vi "Project Documentation 2012 NIVerified.vi"() -> ()   [LabVIEW 2021]
panel:
  out "Project Descriptions":string[](array[string])
  # "Overview: This example uses recursion to harvest and publish documentation for a LabVIEW project.\nRequirements: LabVIEW 2012 (or compatible)\nInstructions:\n1. Open the project(s) you want to document.\n2. Run this VI .\n3. Observe the  Project Descriptions control, it will document all the open projects, and change the index to see\n documentation of different projects."
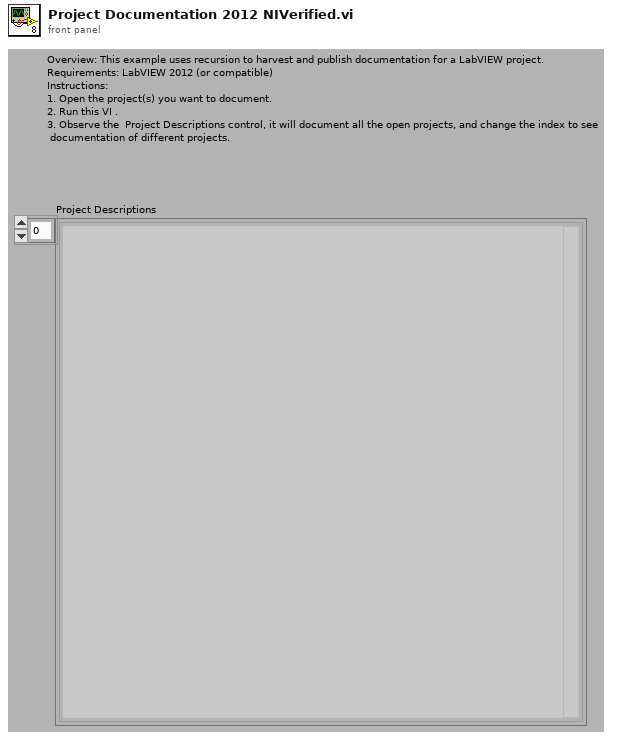
[diagram p1: front panel]
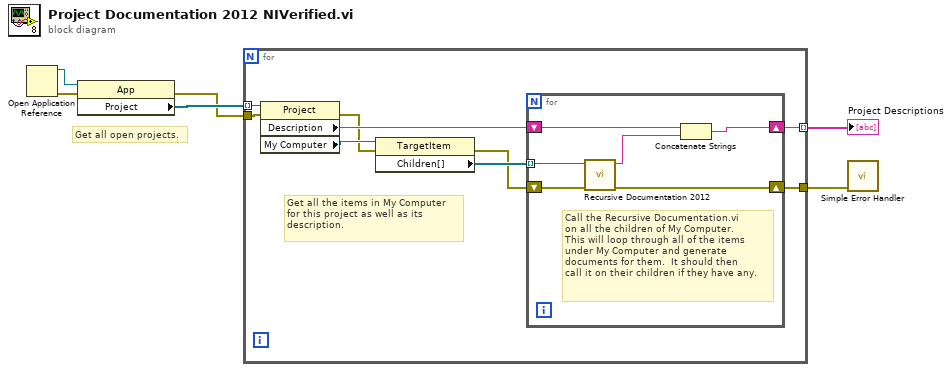
[diagram p0: block diagram]
diagram:
  # "Get all open projects."
  n1 = Open Application Reference() -> (0:w5:errorcluster, 3:w6:refnum<vi>)  [unwired: 4 in]
  n2 = property class="App"(reference=w6, error in=w5) -> (error out=w2:errorcluster, "Project"=w4:refnum<vi>[])  [unwired: 1 out]
  n3 = for {
    tunnel: w4 -> [w11] mode=indexing
    tunnel: [w12] -> w3 mode=indexing
    tunnel: w2 -> [w10]
    tunnel: [w7] -> w1
    # "Get all the items in My Computer\nfor this project as well as its\ndescription."
    n4 = property class="Project"(reference=w11, error in=w10) -> (error out=w9:errorcluster, "Description"=w13:string, "My Computer"=w15:refnum<vi>)  [unwired: 1 out]
    n5 = property class="TargetItem"(reference=w15, error in=w9) -> (error out=w8:errorcluster, "Children[]"=w14:refnum<vi>[])  [unwired: 1 out]
    n6 = for {
      tunnel: w14 -> [w21] mode=indexing
      shift-right: [w18] -> w12
      shift-left: w13 -> [w19]
      shift-right: [w16] -> w7
      shift-left: w8 -> [w20]
      # "Call the Recursive Documentation.vi \non all the children of My Computer.  \nThis will loop through all of the items \nunder My Computer and generate \ndocuments for them.  It should then \ncall it on their children if they have any."
      n7 = call "Recursive Documentation 2012.vi"("error in (no error)"=w20, "Project Item Refnum"=w21) -> ("error IO"=w16:errorcluster, "String"=w17:string)  [unwired: 8 in]
      n8 = Concatenate Strings(w19, w17) -> (w18:string)
    }
  }
  "Project Descriptions" <- w3
  n9 = call <vilib>:"Simple Error Handler.vi"("error in (no error)"=w1) -> ()  [unwired: 4 in, 5 out]
